vi "subDFD_Get Boolean Value by Name.vi"(8 "error in (no error)":errorcluster, 9 "Control Name":string, 11 "vi reference in":refnum<vi>) -> (0 "error out":errorcluster, 1 "Boolean":bool, 3 "vi reference out":refnum<vi>)   [LabVIEW 2023]
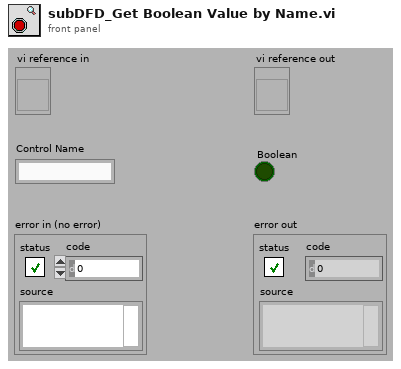
[diagram p1: front panel]
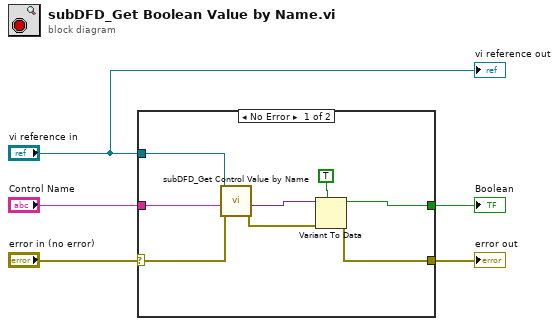
[diagram p0: block diagram]
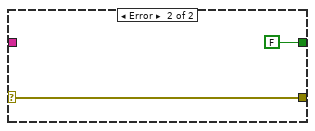
[diagram p2: hidden frame]
diagram:
  n1 = case shown="No Error" "error in (no error)" {
    selector: "error in (no error)" -> [w12 w15]
    tunnel: "vi reference in" -> [w7 _]
    tunnel: "Control Name" -> [w13 _]
    tunnel: [w8 FALSE] -> w3
    tunnel: [w6 w15] -> w2
    frame No Error {
      n2 = call "subDFD_Get Control Value by Name.vi"("error IO"=w12, "Control Name"=w13, "vi reference in"=w7) -> ("error out"=w10:errorcluster, "Value"=w11:variant)  [unwired: 7 out]
      n3 = Variant To Data(error in=w10, type=TRUE, Variant=w11) -> (data=w8:bool, error out=w6:errorcluster)
    }
    frame Error {
    }
  }
  "Boolean" <- w3
  "error out" <- w2
  "vi reference out" <- "vi reference in"
